vi "Leer_propiedades.vi"() -> ()   [LabVIEW 2016]
uses:
  <vilib>/Utility/miscctls.llb/LVPositionTypeDef.ctl
  <vilib>/Utility/miscctls.llb/LVBoundsTypeDef.ctl
panel:
  out "Button Size":T1
  out "Position":T2
  out "Boolean":bool
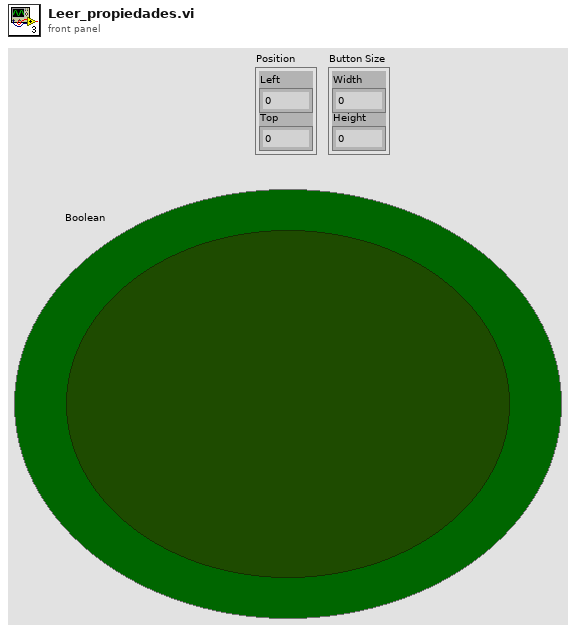
[diagram p1: front panel]
types:
  T1 = typedef "LVBoundsTypeDef.ctl" = cluster{"Width":u32, "Height":u32}
  T2 = typedef "LVPositionTypeDef.ctl" = cluster{"Left":i32, "Top":i32}
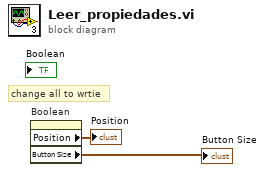
[diagram p0: block diagram]
diagram:
  # "change all to wrtie"
  n1 = property on="Boolean" class="Bool (strict)"() -> ("Position"=→"Position":T2, "Button Size"=→"Button Size":T1)  [unwired: 2 in, 2 out]
